vi "Lift.vi"(11 "Effort":dbl format="%#_13g") -> ()   [LabVIEW 2017]
uses:
  <vilib>/Rock Robotics/WPI/ThirdParty/Phoenix-LabVIEW/Motor Controller/Controls/CTRE_Phoenix_MotorControl_ControlMode.ctl
  UpperSwitchPressed.vi
  LowerSwitchPressed.vi
  <vilib>/Rock Robotics/WPI/ThirdParty/Phoenix-LabVIEW/Motor Controller/Get/CTRE_Phoenix_MotorController_GetQuadratureData.vi
panel:
  out "LiftLower":bool
  out "LiftUpper":bool
  out "LiftVal 2":i32
  out "LiftVal":i32
  in  "Min Joystick":dbl=0.3 format="%#_13g"
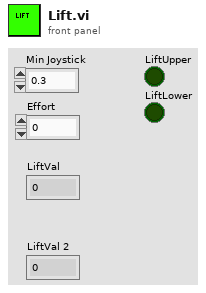
[diagram p1: front panel]
types:
  T1 = typedef "CTRE_Phoenix_MotorControl_ControlMode.ctl" = u16
  T2 = typedef "WPI_MotorControlDeviceRef.ctl" = cluster{"DeviceStatus":errorcluster, "Type":T3, "PWM":cluster{"PWM Channel":T4, "DeadBand":T5}, "CAN":cluster{"Device Number":u8, "SetOutput VI Ref":variant, "GetOutput VI Ref":variant, "Enable VI Ref":variant, "Disable VI Ref":variant, "Data":variant}, "Invert":bool, "DIO PWM":cluster{"PWM \"Enable\" Channel":T4, "DIOChannel":T6, "PWM Rate":dbl}}
  T3 = typedef "WPI_MotorControlType.ctl" = enum16{"PWM", "CAN", "DIO PWM"}
  T4 = typedef "FPGA_DIOPWMChannel.ctl" = enum8{"PWM 0", "PWM 1", "PWM 2", "PWM 3", "PWM 4", "PWM 5", "PWM 6", "PWM 7", "PWM 8", "PWM 9", "PWM MXP 0", "PWM MXP 1", "PWM MXP 2", "PWM MXP 3", "PWM MXP 4", "PWM MXP 5", "PWM MXP 6", "PWM MXP 7", "PWM MXP 8", "PWM MXP 9", "Invalid"}
  T5 = typedef "WPI_PWMDeadband.ctl" = cluster{"Name":string, "maxPositivePwm":i32, "minPositivePwm":i32, "centerPwm":i32, "maxNegativePwm":i32, "minNegativePwm":i32, "angularRange":u16}
  T6 = typedef "FPGA_DIOChannel.ctl" = enum8{"DIO 0", "DIO 1", "DIO 2", "DIO 3", "DIO 4", "DIO 5", "DIO 6", "DIO 7", "DIO 8", "DIO 9", "DIO MXP 0", "DIO MXP 1", "DIO MXP 2", "DIO MXP 3", "DIO MXP 4", "DIO MXP 5", "DIO MXP 6", "DIO MXP 7", "DIO MXP 8", "DIO MXP 9", "DIO MXP 10", "DIO MXP 11", "DIO MXP 12", "DIO MXP 13", "DIO MXP 14", "DIO MXP 15", "SPI Port CS1", "SPI Port CS2", "SPI Port CS3", "SPI Port MISO", "SPI Port MOSI", "Invalid"}
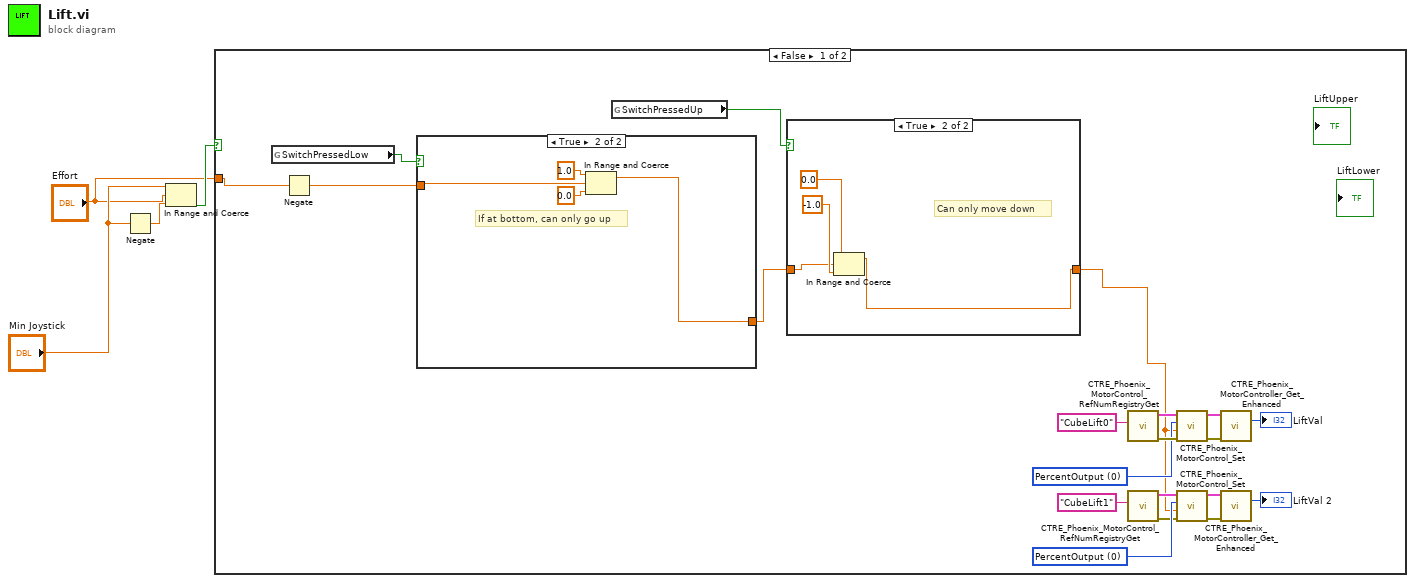
[diagram p0: block diagram]
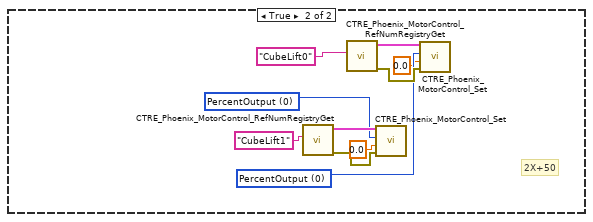
[diagram p4: hidden frame]
diagram:
  n1 = Negate(x="Min Joystick") -> (-x=w3:dbl)
  n2 = In Range and Coerce(upper limit="Min Joystick", x="Effort", lower limit=w3) -> (In Range?=w2:bool)  [unwired: 1 out]
  n3 = case shown="False" w2 {
    tunnel: "Effort" -> [w20 _]
    frame False {
      w13 = T1 0 items=["PercentOutput"=0, "Position"=1, "Velocity"=2, "Current"=3, "Follower"=5, "MotionProfile"=6, "MotionMagic"=7, "MotionMagicArc"=8, "MotionProfileArc"=10, "Disabled"=15] ("Control Mode")
      w21 = T1 0 items=["PercentOutput"=0, "Position"=1, "Velocity"=2, "Current"=3, "Follower"=5, "MotionProfile"=6, "MotionMagic"=7, "MotionMagicArc"=8, "MotionProfileArc"=10, "Disabled"=15] ("Control Mode")
      n4 = global read "LowerSwitchPressed.vi" "SwitchPressedLow"() -> (w6:bool)
      n5 = Negate(x=w20) -> (-x=w8:dbl)
      n6 = case shown="True" w6 {
        tunnel: w8 -> [w30 w33]
        tunnel: [w30 w31] -> w7
        frame False {
          # "If not at bottom, can move either way"
        }
        frame True {
          # "If at bottom, can only go up"
          n7 = In Range and Coerce(upper limit=1.0, x=w33, lower limit=0.0) -> (coerced(x)=w31:dbl)  [unwired: 1 out]
        }
      }
      n8 = global read "UpperSwitchPressed.vi" "SwitchPressedUp"() -> (w5:bool)
      n9 = case shown="True" w5 {
        tunnel: [w25 w27] -> w9
        tunnel: w7 -> [w25 w26]
        frame False {
        }
        frame True {
          # "Can only move down"
          n10 = In Range and Coerce(upper limit=0.0, x=w26, lower limit=-1.0) -> (coerced(x)=w27:dbl)  [unwired: 1 out]
        }
      }
      n11 = call <vilib>:"CTRE_Phoenix_MotorControl_RefNumRegistryGet.vi"("refnum name"="CubeLift0") -> ("error out"=w23:errorcluster, "PhoenixMotorControlDevRef"=w24:T2)  [unwired: 9 in]
      n12 = call <vilib>:"CTRE_Phoenix_MotorControl_RefNumRegistryGet.vi"("refnum name"="CubeLift1") -> ("error out"=w11:errorcluster, "PhoenixMotorControlDevRef"=w10:T2)  [unwired: 9 in]
      n13 = call <vilib>:"CTRE_Phoenix_MotorControl_Set.vi"("error in (no error)"=w23, "Output"=w9, "Control Mode"=w21, "PhoenixMotorControlDevRef"=w24) -> ("error out"=w18:errorcluster, "PhoenixMotorControlDevRef"=w19:T2)  [unwired: 6 in]
      n14 = call <vilib>:"CTRE_Phoenix_MotorControl_Set.vi"("error in (no error)"=w11, "Output"=w9, "Control Mode"=w13, "PhoenixMotorControlDevRef"=w10) -> ("error out"=w15:errorcluster, "PhoenixMotorControlDevRef"=w14:T2)  [unwired: 6 in]
      n15 = call-poly <vilib>:"CTRE_Phoenix_MotorController_Get_Enhanced.vi"("PhoenixMotorControlDevRef"=w19, "error in"=w18) -> ("Quadrature Position"=→"LiftVal":i32)  [unwired: 10 in, 3 out]
      n16 = call-poly <vilib>:"CTRE_Phoenix_MotorController_Get_Enhanced.vi"("PhoenixMotorControlDevRef"=w14, "error in"=w15) -> ("Quadrature Position"=→"LiftVal 2":i32)  [unwired: 10 in, 3 out]
    }
    frame True {
      w37 = T1 0 items=["PercentOutput"=0, "Position"=1, "Velocity"=2, "Current"=3, "Follower"=5, "MotionProfile"=6, "MotionMagic"=7, "MotionMagicArc"=8, "MotionProfileArc"=10, "Disabled"=15] ("Control Mode")
      w41 = T1 0 items=["PercentOutput"=0, "Position"=1, "Velocity"=2, "Current"=3, "Follower"=5, "MotionProfile"=6, "MotionMagic"=7, "MotionMagicArc"=8, "MotionProfileArc"=10, "Disabled"=15] ("Control Mode")
      # "2X+50"
      n17 = call <vilib>:"CTRE_Phoenix_MotorControl_RefNumRegistryGet.vi"("refnum name"="CubeLift1") -> ("error out"=w40:errorcluster, "PhoenixMotorControlDevRef"=w39:T2)  [unwired: 9 in]
      n18 = call <vilib>:"CTRE_Phoenix_MotorControl_RefNumRegistryGet.vi"("refnum name"="CubeLift0") -> ("error out"=w44:errorcluster, "PhoenixMotorControlDevRef"=w43:T2)  [unwired: 9 in]
      n19 = call <vilib>:"CTRE_Phoenix_MotorControl_Set.vi"("error in (no error)"=w40, "Output"=0.0, "Control Mode"=w37, "PhoenixMotorControlDevRef"=w39) -> ()  [unwired: 6 in, 2 out]
      n20 = call <vilib>:"CTRE_Phoenix_MotorControl_Set.vi"("error in (no error)"=w44, "Output"=0.0, "Control Mode"=w41, "PhoenixMotorControlDevRef"=w43) -> ()  [unwired: 6 in, 2 out]
    }
  }
